vi "Check image quality.vi"(8 "error in (no error)":errorcluster, 11 "Cascade in":refnum<class "Cascade.lvclass">) -> (0 "error out":errorcluster, 2 "QC passed?":bool, 3 "Cascade out":refnum<class "Cascade.lvclass">)   [LabVIEW 2012, in "Cascade.lvclass"]
uses:
  Cascade.lvclass
  Cascade.lvclass/Cascade.ctl
  <vilib>/vision/NI_Vision_Development_Module.lvlib
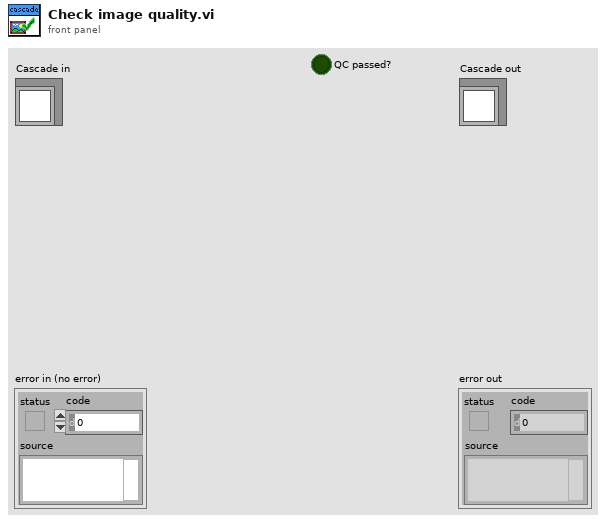
[diagram p1: front panel]
types:
  T1 = typedef "IMAQ Image.ctl" = refnum<image>
  T2 = cluster{"histogram":u32[], "Minimal Value":sgl, "Maximal Value":sgl, "Starting Value":sgl, "Interval Width":sgl, "Mean Value":sgl, "Standard  Variation":sgl, "Area (pixels)":i32}
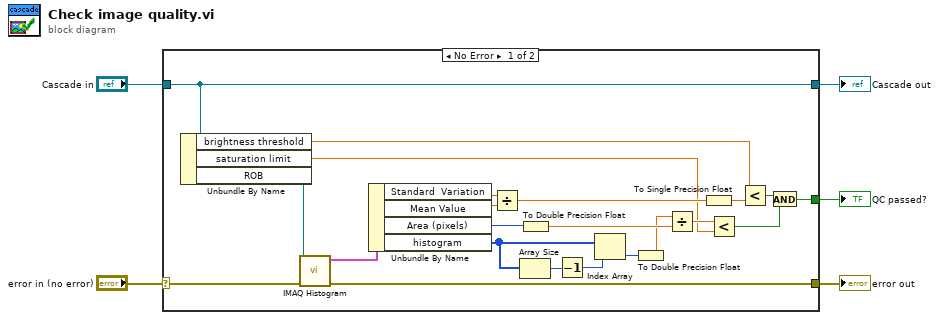
[diagram p0: block diagram]
diagram:
  n1 = case shown="No Error" "error in (no error)" {
    selector: "error in (no error)" -> [w12 w29]
    tunnel: [w11 w29] -> w4
    tunnel: [w10 w28] -> w2
    tunnel: "Cascade in" -> [w10 w28]
    tunnel: [w6 _] -> w1
    frame No Error {
      n2 = Unbundle By Name(w10) -> ("brightness threshold"=w7:sgl, "saturation limit"=w8:dbl, "ROB"=w9:T1)
      n3 = call "IMAQ Histogram"("error in (no error)"=w12, "Image"=w9) -> ("error out"=w11:errorcluster, "Histogram Report"=w26:T2)  [unwired: 8 in]
      n4 = Unbundle By Name(w26) -> ("Standard  Variation"=w25:sgl, "Mean Value"=w24:sgl, "Area (pixels)"=w19:i32, "histogram"=w22:u32[])
      n5 = Divide(x=w25, y=w24) -> (x/y=w23:sgl)
      n6 = Array Size(array=w22) -> (size(s)=w21:i32)
      n7 = To Double Precision Float(number=w19) -> (double precision float=w17:dbl)
      n8 = Decrement(x=w21) -> (x-1=w20:i32)
      n9 = Index Array(array=w22, index=w20) -> (element=w18:u32)
      n10 = To Double Precision Float(number=w18) -> (double precision float=w15:dbl)
      n11 = Divide(x=w15, y=w17) -> (x/y=w16:dbl)
      n12 = To Single Precision Float(number=w23) -> (single precision float=w27:sgl)
      n13 = Less?(x=w16, y=w8) -> (x < y?=w14:bool)
      n14 = Less?(x=w7, y=w27) -> (x < y?=w13:bool)
      n15 = And(x=w13, y=w14) -> (x .and. y?=w6:bool)
    }
    frame Error {
    }
  }
  "error out" <- w4
  "Cascade out" <- w2
  "QC passed?" <- w1
